vi "3dLoad.vi"(11 "name or relative path":string="..\\Hexa1.stl") -> (0 "Object":refnum<vi>, 1 "reference out":refnum<vi>, 3 "appended path 2":path)   [LabVIEW 2011]
uses:
  <vilib>/picture/3D Picture Control/NI_3D Picture Control.lvlib
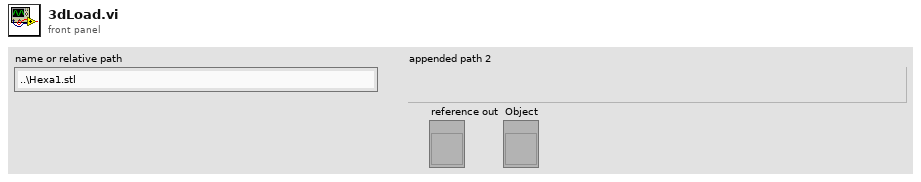
[diagram p1: front panel]
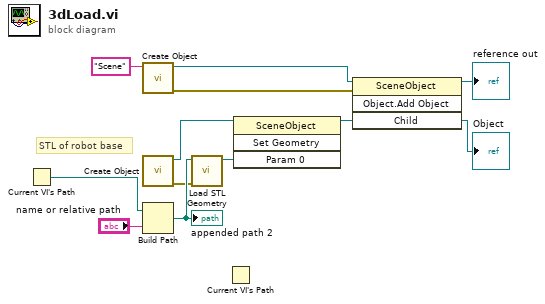
[diagram p0: block diagram]
diagram:
  # "STL of robot base"
  n1 = Current VI's Path() -> (path=w8:path)
  n2 = call <vilib>:"Create Object.vi"("Name"="Scene") -> ("error out"=w12:errorcluster, "Scene:New Object"=w11:refnum<vi>)  [unwired: 9 in]
  n3 = call <vilib>:"Create Object.vi"() -> ("error out"=w5:errorcluster, "Scene:New Object"=w6:refnum<vi>)  [unwired: 10 in]
  n4 = Build Path(base path=w8, name or relative path="name or relative path") -> (appended path=w9:path)
  "appended path 2" <- w9
  n5 = call <vilib>:"Load STL Geometry.vi"("error in (no error)"=w5, "Model File"=w9) -> ("New Mesh Refnum"=w7:refnum<vi>)  [unwired: 8 in, 1 out]
  n6 = Current VI's Path() -> ()  [unwired: 1 out]
  n7 = invoke class="SceneObject" method="Set Geometry"(reference=w6, "Param 0"=w7) -> (reference out=w4:refnum<vi>)  [unwired: 2 in, 3 out]
  n8 = invoke class="SceneObject" method="Object.Add Object"(reference=w11, error in=w12, "Child"=w4) -> (reference out=→"reference out":refnum<vi>, "Child"=→"Object":refnum<vi>)  [unwired: 1 in, 2 out]
